vi "Update Set Membership.vi"(10 "node ref in":refnum<data-value>, 11 "AD* in":refnum<class "NI_Robotics_AnytimeDStar.lvclass">) -> (2 "node ref out":refnum<data-value>, 3 "AD* out":refnum<class "NI_Robotics_AnytimeDStar.lvclass">)   [LabVIEW 2017, in "NI_Robotics_AnytimeDStar.lvclass"]
uses:
  <vilib>/robotics/Navigation/Anytime D Star/NI_Robotics_AnytimeDStar.lvclass
  <vilib>/robotics/Navigation/shared/MapNode/AbstractDstarNode/NI_Robotics_AbstractDstarNode.lvclass
  c:/Program Files (x86)/National Instruments/LabVIEW 2017/vi.lib/robotics/Navigation/shared/MapNode/AbstractMapNode/NI_Robotics_AbstractMapNode.lvclass
  <vilib>/robotics/Navigation/Anytime D Star/NI_Robotics_AnytimeDStar.lvclass/NI_Robotics_AnytimeDStar.ctl
  <vilib>/robotics/Navigation/shared/Priority Queue/NI_Robotics_Priority Queue.lvclass
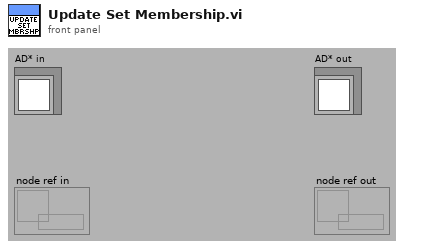
[diagram p1: front panel]
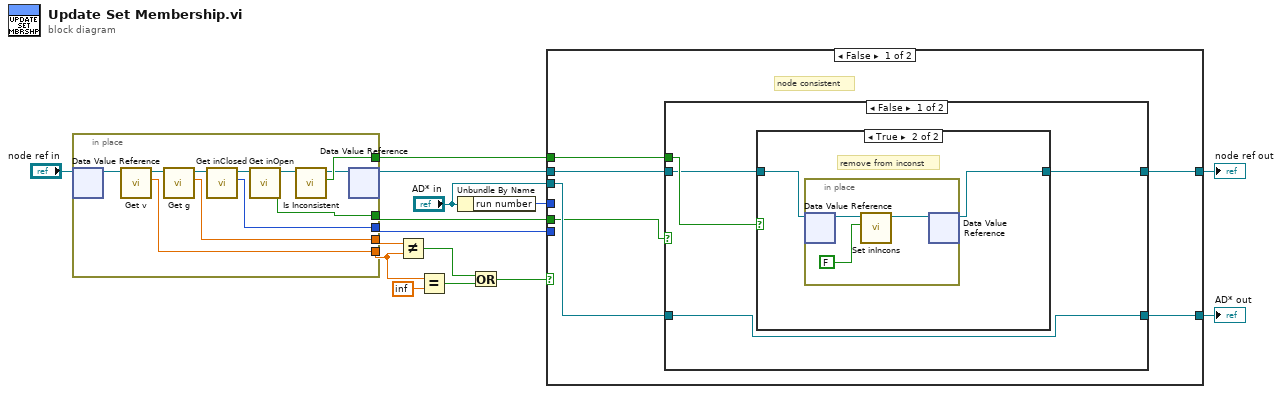
[diagram p0: block diagram]
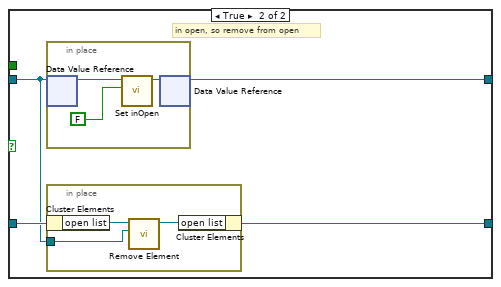
[diagram p3: hidden frame]
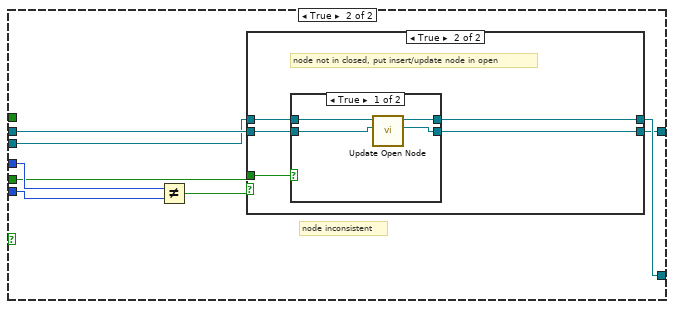
[diagram p4: hidden frame]
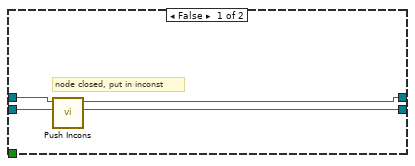
[diagram p5: hidden frame]
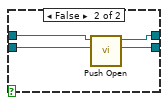
[diagram p6: hidden frame]
diagram:
  n1 = in-place {
    in-place-border: [w23] -> w14
    in-place-border: [w22] -> w5
    in-place-border: [w21] -> w4
    in-place-border: [w19] -> w3
    in-place-border: [w17] -> w1
    n2 = in-place-dvr #1("node ref in") -> (w26:refnum<class "NI_Robotics_AbstractDstarNode.lvclass">)  [unwired: 1 out]
    n3 = call <vilib>:"Get v.vi"("AbstractDstarNode in"=w26) -> ("v"=w21:dbl, "AbstractDstarNode out"=w25:refnum<class "NI_Robotics_AbstractDstarNode.lvclass">)  [unwired: 9 in]
    n4 = call <vilib>:"Get g.vi"("AbstractDstarNode in"=w25) -> ("g"=w22:dbl, "AbstractDstarNode out"=w24:refnum<class "NI_Robotics_AbstractDstarNode.lvclass">)  [unwired: 9 in]
    n5 = call <vilib>:"Get inClosed.vi"("AbstractDstarNode in"=w24) -> ("inClosed"=w23:i32, "AbstractDstarNode out"=w20:refnum<class "NI_Robotics_AbstractDstarNode.lvclass">)  [unwired: 8 in, 1 out]
    n6 = call <vilib>:"Get inOpen.vi"("AbstractDstarNode in"=w20) -> ("inOpen"=w19:bool, "AbstractDstarNode out"=w18:refnum<class "NI_Robotics_AbstractDstarNode.lvclass">)  [unwired: 8 in, 1 out]
    n7 = call <vilib>:"Is Inconsistent.vi"("AbstractDstarNode in"=w18) -> ("is Inconsistent"=w17:bool, "AbstractDstarNode out"=w16:refnum<class "NI_Robotics_AbstractDstarNode.lvclass">)  [unwired: 8 in, 1 out]
    n8 = in-place-dvr #1(w16) -> (w12:refnum<data-value>)  [unwired: 1 out]
  }
  n9 = Not Equal?(x=w5, y=w4) -> (x != y?=w9:bool)
  n10 = Equal?(x=w4, y=inf) -> (x = y?=w7:bool)
  n11 = Unbundle By Name("AD* in") -> ("run number"=w13:i32)
  n12 = Or(x=w9, y=w7) -> (x .or. y?=w8:bool)
  n13 = case shown="False" w8 {
    tunnel: [w30 w59] -> w2
    tunnel: w14 -> [_ w58]
    tunnel: w13 -> [_ w57]
    tunnel: w12 -> [w29 w56]
    tunnel: "AD* in" -> [w31 w55]
    tunnel: [w32 w54] -> w10
    tunnel: w3 -> [w28 w53]
    tunnel: w1 -> [w27 _]
    frame False {
      # "node consistent"
      n14 = case shown="False" w28 {
        tunnel: [w33 w46] -> w32
        tunnel: w31 -> [w34 w45]
        tunnel: [w34 w44] -> w30
        tunnel: w29 -> [w35 w43]
        tunnel: w27 -> [w36 _]
        frame False {
          n15 = case shown="True" w36 {
            tunnel: w35 -> [w37 w39]
            tunnel: [w37 w38] -> w33
            frame False {
            }
            frame True {
              # "remove from inconst"
              n16 = in-place {
                n17 = in-place-dvr #2(w39) -> (w40:refnum<class "NI_Robotics_AbstractDstarNode.lvclass">)  [unwired: 1 out]
                n18 = call <vilib>:"Set inIncons.vi"("inIncons"=FALSE ("inOpen"), "AbstractDstarNode in"=w40) -> ("AbstractDstarNode out"=w42:refnum<class "NI_Robotics_AbstractDstarNode.lvclass">)  [unwired: 9 in]
                n19 = in-place-dvr #2(w42) -> (w38:refnum<data-value>)  [unwired: 1 out]
              }
            }
          }
        }
        frame True {
          # "in open, so remove from open"
          n20 = in-place {
            n21 = in-place-dvr #3(w43) -> (w50:refnum<class "NI_Robotics_AbstractDstarNode.lvclass">)  [unwired: 1 out]
            n22 = call <vilib>:"Set inOpen.vi"("inOpen"=FALSE, "AbstractDstarNode in"=w50) -> ("AbstractDstarNode out"=w52:refnum<class "NI_Robotics_AbstractDstarNode.lvclass">)  [unwired: 8 in, 1 out]
            n23 = in-place-dvr #3(w52) -> (w46:refnum<data-value>)  [unwired: 1 out]
          }
          n24 = in-place {
            in-place-border: w43 -> [w47]
            n25 = in-place-cluster #4(w45) -> ("open list"=w48:refnum<class "NI_Robotics_Priority Queue.lvclass">)
            n26 = call <vilib>:"Remove Element.vi"("node Ref"=w47, "Priority Queue in"=w48) -> ("Priority Queue out"=w49:refnum<class "NI_Robotics_Priority Queue.lvclass">)  [unwired: 8 in, 1 out]
            n27 = in-place-cluster #4("open list"=w49) -> (w44:refnum<class "NI_Robotics_AnytimeDStar.lvclass">)
          }
        }
      }
    }
    frame True {
      # "node inconsistent"
      n28 = Not Equal?(x=w57, y=w58) -> (x != y?=w60:bool)
      n29 = case shown="True" w60 {
        tunnel: [w64 w69] -> w59
        tunnel: w56 -> [w62 w68]
        tunnel: w55 -> [w63 w67]
        tunnel: [w61 w66] -> w54
        tunnel: w53 -> [_ w65]
        frame False {
          # "node closed, put in inconst"
          n30 = call <vilib>:"Push Incons.vi"("node ref in"=w62, "adstar in"=w63) -> ("node ref out"=w61:refnum<data-value>, "adstar out"=w64:refnum<class "NI_Robotics_AnytimeDStar.lvclass">)  [unwired: 8 in]
        }
        frame True {
          # "node not in closed, put insert/update node in open"
          n31 = case shown="True" w65 {
            tunnel: [w71 w77] -> w69
            tunnel: w68 -> [w72 w76]
            tunnel: w67 -> [w73 w75]
            tunnel: [w70 w74] -> w66
            frame True {
              n32 = call <vilib>:"Update Open Node.vi"("node ref in"=w72, "AD* in"=w73) -> ("node ref out"=w70:refnum<data-value>, "AD* out"=w71:refnum<class "NI_Robotics_AnytimeDStar.lvclass">)  [unwired: 8 in]
            }
            frame False {
              n33 = call <vilib>:"Push Open.vi"("node ref in"=w76, "AD* in"=w75) -> ("node ref out"=w74:refnum<data-value>, "AD* out"=w77:refnum<class "NI_Robotics_AnytimeDStar.lvclass">)  [unwired: 8 in]
            }
          }
        }
      }
    }
  }
  "AD* out" <- w2
  "node ref out" <- w10
